vi "Set_RAW_Array.vi"(0 "reference in":refnum<class "AI.lvclass">, 5 "RAW":dbl[](array[numeric]), 11 "error in (no error)":errorcluster) -> (4 "reference out":refnum<class "AI.lvclass">, 15 "error out":errorcluster)   [LabVIEW 2019, in "AI.lvclass"]
uses:
  AI.lvclass
  AI.lvclass/AI.ctl
  PiecedLinearScale_class/Scale_PiecedLinear.lvclass/Scale_PiecedLinear.ctl
  AnalogComparator_class/AnalogComparator.lvclass/AnalogComparator.ctl
  PiecedLinearScale_class/RawToScaled.vi
  HandleRanges.vi
  HandleAlarms.vi
  AnalogComparator_class/SetValue.vi
  <vilib>/gmath/interp.llb/Interpolate 1D.vi
  <vilib>/Utility/error.llb/Error Cluster From Error Code.vi
  subvis/Average.vi
  AnalogComparator_class/HandleDb.vi
  <vilib>/Analysis/NI_AALBase.lvlib
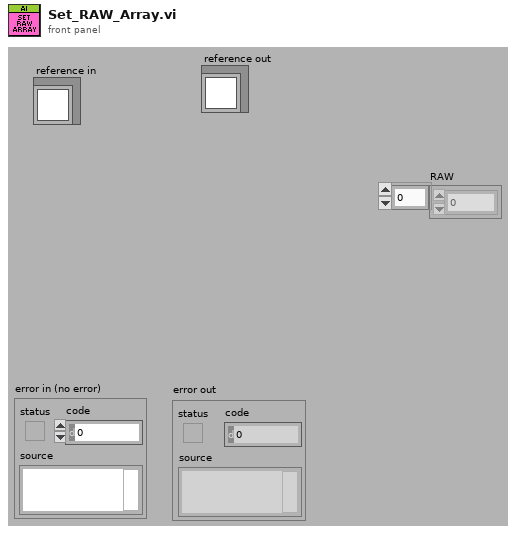
[diagram p1: front panel]
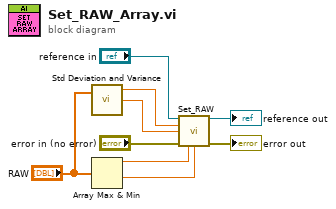
[diagram p0: block diagram]
diagram:
  n1 = call <vilib>:"Std Deviation and Variance.vi"("X"="RAW") -> ("mean"=w2:dbl, "standard deviation"=w1:dbl)  [unwired: 1 in, 1 out]
  n2 = Array Max & Min(array="RAW") -> (max value=w4:dbl, min value=w3:dbl)  [unwired: 2 out]
  n3 = call "Set_RAW.vi"("reference in"="reference in", "raw mean"=w2, "raw standard deviation"=w1, "error in (no error)"="error in (no error)", "raw max value"=w4, "raw min value"=w3) -> ("reference out"=→"reference out":refnum<class "AI.lvclass">, "error out"=→"error out":errorcluster)  [unwired: 8 in]
